vi "Anritsu VNA Set Cal Off.vi"(7 "Anritsu VNA":T1, 8 "error in (no error)":errorcluster, 11 "VISA Resource Name":refnum<visa-resource-name>) -> (0 "error out":errorcluster {"code" format="%.0x"}, 3 "dup VISA Resource Name":refnum<visa-resource-name>)   [LabVIEW 2011]
doc: "This Vi for the HP8753B Network Analyzer is used to set averaging, smoothing, and the IF bandwidth."
uses:
  TypeDefs/Anritsu VNA Instrument Info.ctl
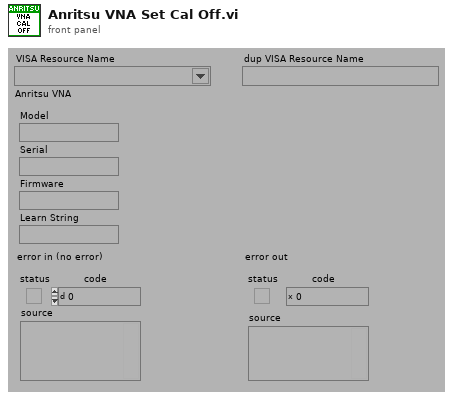
[diagram p1: front panel]
types:
  T1 = typedef "Anritsu VNA Instrument Info.ctl" = cluster{"Model":string, "Serial":string, "Firmware":string, "Learn String":string}
  T2 = typedef "Anritsu VNA Model.ctl" = enum16{"Not Supported", "37XXXX", "MS20XXX", "MS462XX", "MS464XX"}
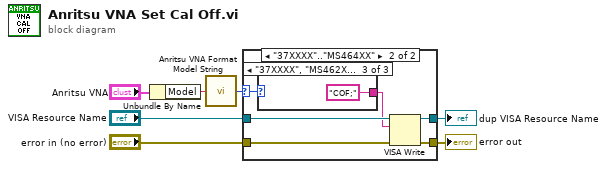
[diagram p0: block diagram]
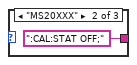
[diagram p4: hidden frame]
diagram:
  n1 = Unbundle By Name("Anritsu VNA") -> ("Model"=w1:string)
  n2 = call "Anritsu VNA Format Model String.vi"("Model"=w1) -> ("Model"=w2:T2)
  n3 = case shown="\"37XXXX\"..\"MS464XX\"" w2 {
    selector: w2 -> [_ w10]
    tunnel: "VISA Resource Name" -> [w9 w15]
    tunnel: "error in (no error)" -> [w8 w14]
    tunnel: [w8 w13] -> w5
    tunnel: [w9 w12] -> w4
    frame "Not Supported" {
    }
    frame "37XXXX".."MS464XX" {
      n4 = case shown="\"37XXXX\", \"MS462XX\", \"MS464XX\"" w10 {
        tunnel: [_ ":CAL:STAT OFF;" "COF;"] -> w11
        frame "Not Supported" {
        }
        frame "MS20XXX" {
        }
        frame "37XXXX", "MS462XX", "MS464XX" {
        }
      }
      n5 = VISA Write(VISA resource name=w15, write buffer=w11, error in (no error)=w14) -> (VISA resource name out=w12:refnum<visa-resource-name>, error out=w13:errorcluster)  [unwired: 1 out]
    }
  }
  "error out" <- w5
  "dup VISA Resource Name" <- w4
